vi "SyncronousLockin_single.vi"(4 "Lock-in settings":T1={"Averaging period, s"=0.0, "Output Representation"=enum."Real/Imaginary", "Output value"=enum."RMS", "Phase delay, points"=0} {"Averaging period, s" format="%#_6p"}, 5 "Raw points to average":i32, 6 "First chunk?":bool, 7 "CH name                          points   phase":T2, 8 "error in (no error)":errorcluster, 11 "Data":waveform(dbl)={"t0"=timestamp(0 s since 1904-01-01), "dt"=0.0, "Y"=[]}) -> (0 "error out":errorcluster, 3 "signal(s) out":waveform(dbl)[](array[waveform]))   [LabVIEW 2015]
uses:
  CH_name_pts_phase.ctl
  Syncronous Lockin Settings.ctl
  <vilib>/measure/NI_MABase.lvlib
panel:
  out "Waveform Graph":waveform(dbl)(graph)
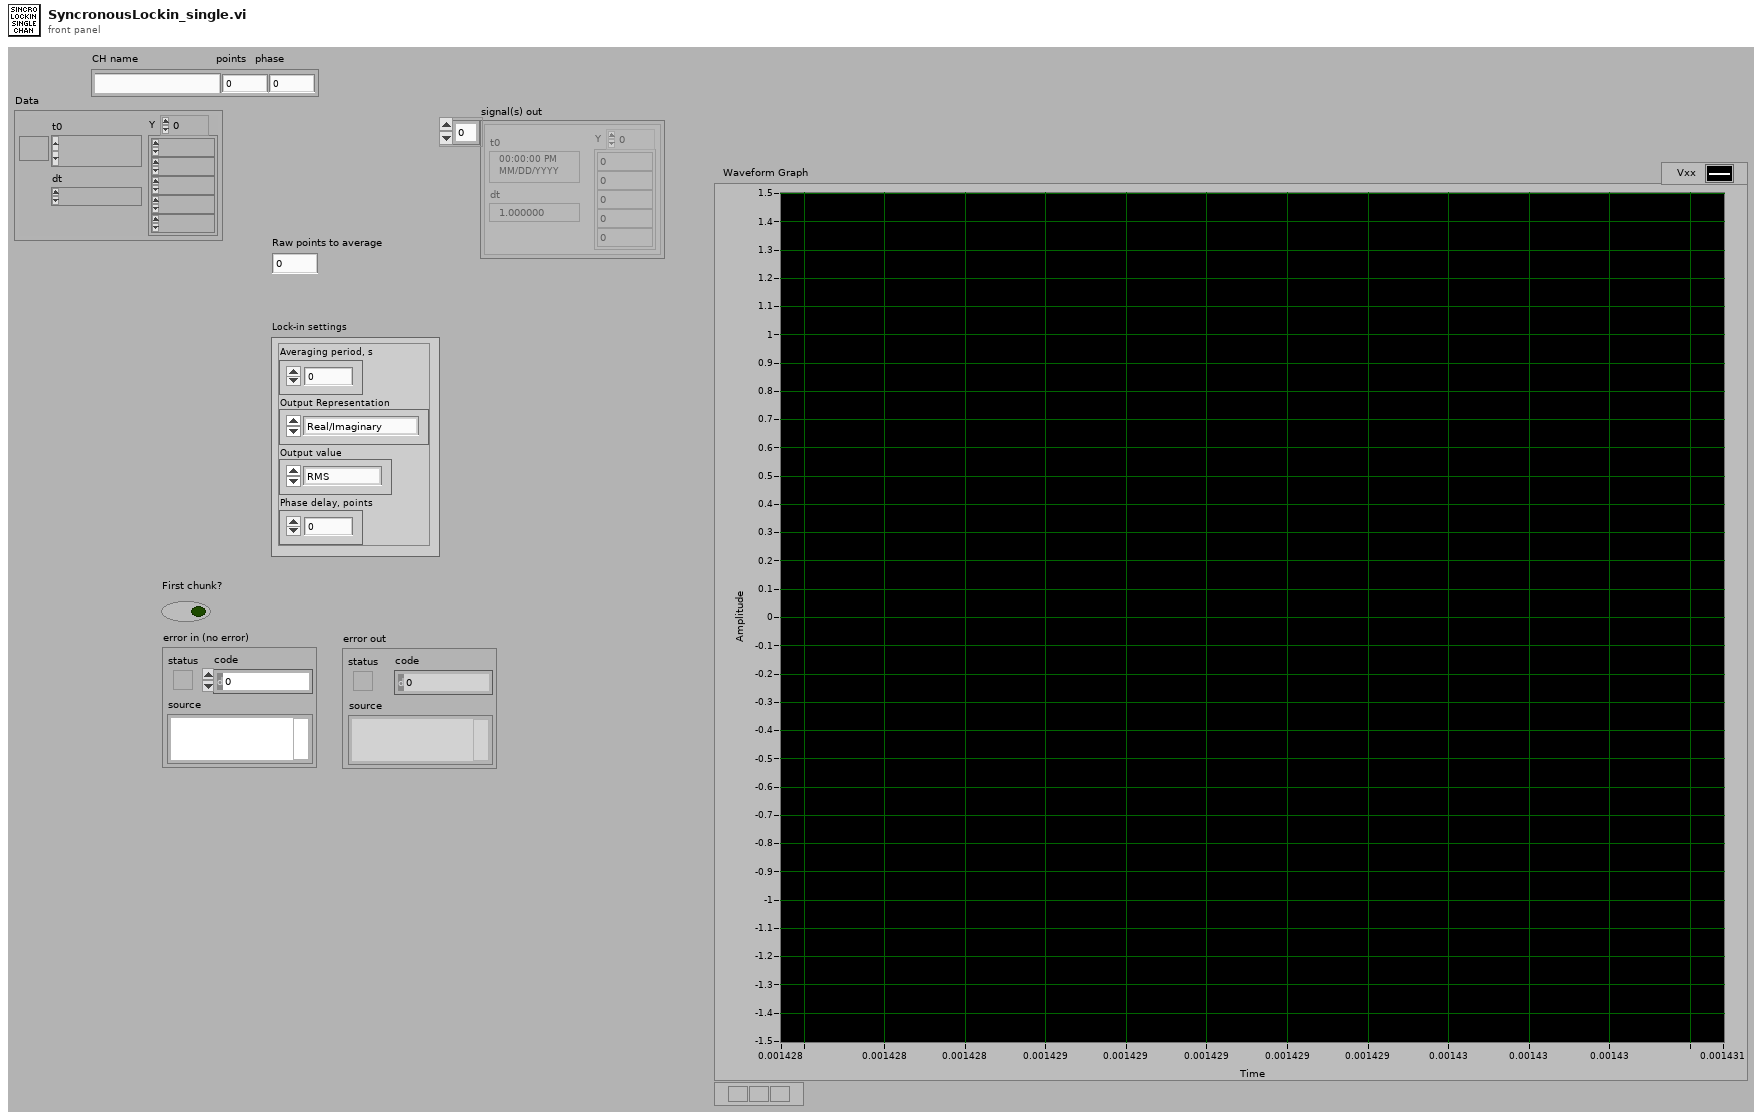
[diagram p1: front panel]
types:
  T1 = typedef "Syncronous Lockin Settings.ctl" = cluster{"Averaging period, s":dbl, "Output Representation":enum16{"Real/Imaginary", "Polar"}, "Output value":enum16{"Amplitude", "RMS", "Peak-to-Peak"}, "Phase delay, points":i32}
  T2 = typedef "CH_name_pts_phase.ctl" = cluster{"Channel":string, "pts per sine wave":i32, "Phase":dbl}
  T3 = enum16{"coerce", "linear", "spline", "Min-Max", "Average"}
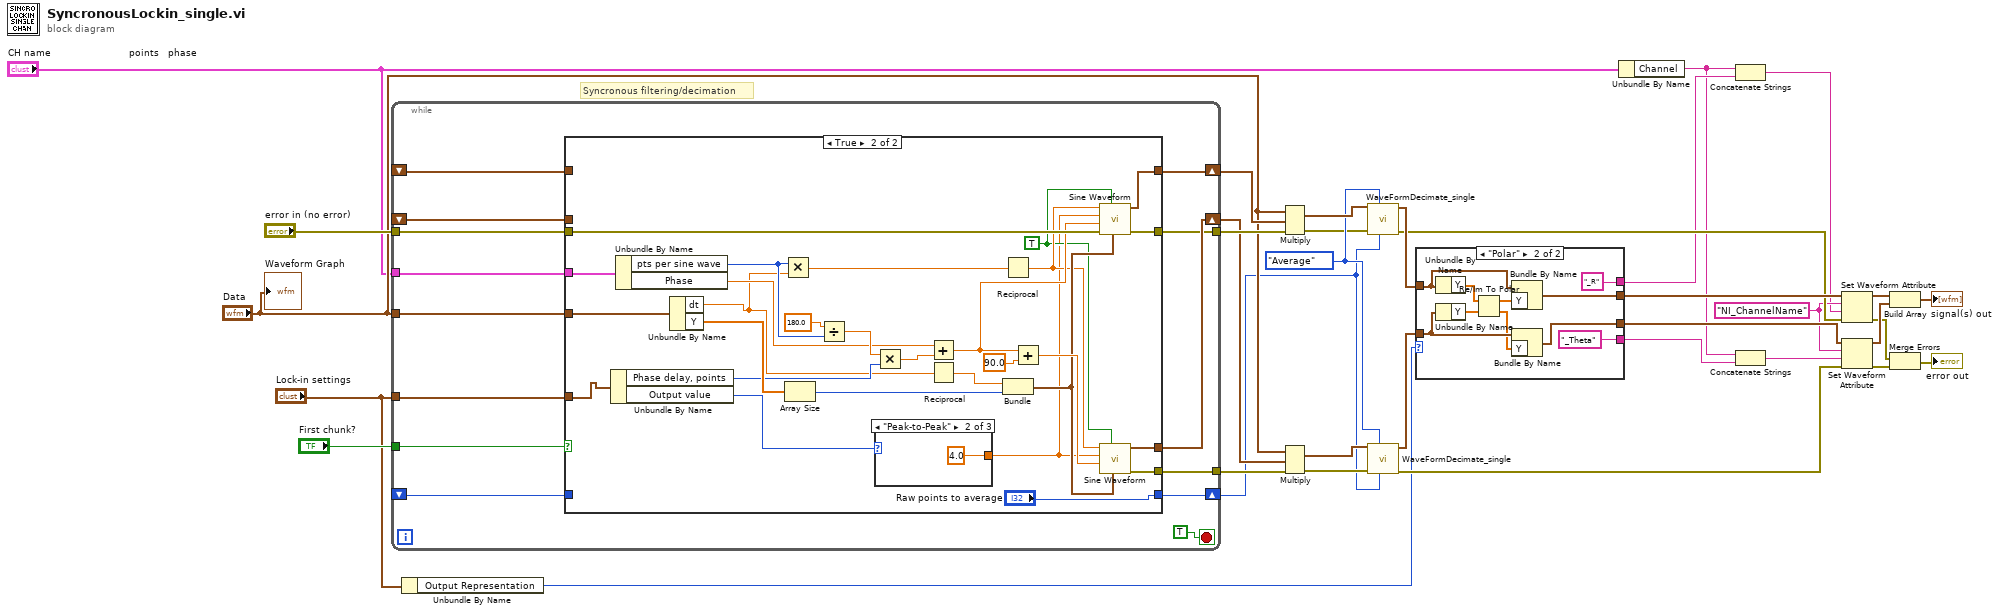
[diagram p0: block diagram]
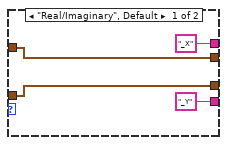
[diagram p2: hidden frame]
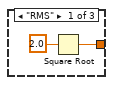
[diagram p4: hidden frame]
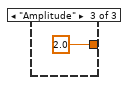
[diagram p5: hidden frame]
diagram:
  w10 = "NI_ChannelName" ("name")
  w24 = T3."Average" ("Plot interpolation")
  # "Syncronous filtering/decimation"
  n1 = while {
    tunnel: "Data" -> [w46]
    tunnel: "error in (no error)" -> [w45]
    tunnel: [w40] -> w33
    shift-right: [w48] -> w31
    shift-left: _ -> [w41]
    shift-right: [w47] -> w30
    shift-left: _ -> [w42]
    tunnel: "First chunk?" -> [w43]
    tunnel: [w39] -> w22
    tunnel: "CH name                          points   phase" -> [w38]
    tunnel: "Lock-in settings" -> [w37]
    shift-right: [w36] -> w3
    shift-left: _ -> [w35]
    stop <- TRUE stop-if-true
    n2 = case shown="True" w43 {
      tunnel: [w51 w79] -> w48
      tunnel: [w52 w78] -> w47
      tunnel: w46 -> [_ w61]
      tunnel: w45 -> [w50 w72]
      tunnel: [w50 w71] -> w39
      tunnel: w42 -> [w52 _]
      tunnel: w41 -> [w51 _]
      tunnel: [w50 w62] -> w40
      tunnel: w38 -> [_ w55]
      tunnel: w37 -> [_ w54]
      tunnel: [w49 "Raw points to average"] -> w36
      tunnel: w35 -> [w49 _]
      frame False {
      }
      frame True {
        w65 = TRUE ("reset signal")
        n3 = Unbundle By Name(w54) -> ("Phase delay, points"=w58:i32, "Output value"=w57:enum16{"Amplitude", "RMS", "Peak-to-Peak"})
        n4 = Unbundle By Name(w55) -> ("pts per sine wave"=w59:i32, "Phase"=w60:dbl)
        n5 = Unbundle By Name(w61) -> ("dt"=w56:dbl, "Y"=w75:dbl[])
        n6 = Multiply(x=w59, y=w56) -> (x*y=w69:dbl)
        n7 = Array Size(array=w75) -> (size(s)=w76:i32)
        n8 = Divide(x=180.0, y=w59) -> (x/y=w67:dbl)
        n9 = Multiply(x=w67, y=w58) -> (x*y=w66:dbl)
        n10 = case shown="\"Peak-to-Peak\"" w57 {
          tunnel: [w81 4.0 ("1/x") 2.0 ("1/x")] -> w63
          frame "RMS" {
            n11 = Square Root(x=2.0 ("1/x")) -> (sqrt(x)=w81:dbl)
          }
          frame "Peak-to-Peak" {
          }
          frame "Amplitude" {
          }
        }
        n12 = Add(x=w60, y=w66) -> (x+y=w70:dbl)
        n13 = Reciprocal(x=w56) -> (1/x=w73:dbl)
        n14 = Reciprocal(x=w69) -> (1/x=w68:dbl)
        n15 = Bundle(w73, w76) -> (w74:cluster{dbl, i32})  [unwired: 1 out]
        n16 = Add(x=w70, y=90.0) -> (x+y=w77:dbl)
        n17 = call <vilib>:"Sine Waveform.vi"("sampling info"=w74, "reset signal"=w65, "error in (no error)"=w72, "phase"=w70, "amplitude"=w63, "frequency"=w68) -> ("error out"=w62:errorcluster, "signal out"=w78:waveform(dbl))  [unwired: 1 in, 3 out]
        n18 = call <vilib>:"Sine Waveform.vi"("sampling info"=w74, "reset signal"=w65, "phase"=w77, "amplitude"=w63, "frequency"=w68) -> ("error out"=w71:errorcluster, "signal out"=w79:waveform(dbl))  [unwired: 2 in, 3 out]
      }
    }
  }
  n19 = Unbundle By Name("Lock-in settings") -> ("Output Representation"=w1:enum16{"Real/Imaginary", "Polar"})
  n20 = Multiply(1:w30, 2:"Data", 4:w33) -> (0:w29:waveform(dbl), 3:w20:errorcluster)
  n21 = Multiply(1:w31, 2:"Data", 4:w22) -> (0:w27:waveform(dbl), 3:w21:errorcluster)
  n22 = call "WaveFormDecimate_single.vi"("Decimation factor"=w3, "Plot interpolation"=w24, "error in (no error)"=w20, "Waveform in"=w29) -> ("error out"=w19:errorcluster, "Waveform out"=w28:waveform(dbl))  [unwired: 6 in]
  n23 = call "WaveFormDecimate_single.vi"("Decimation factor"=w3, "Plot interpolation"=w24, "error in (no error)"=w21, "Waveform in"=w27) -> ("error out"=w14:errorcluster, "Waveform out"=w26:waveform(dbl))  [unwired: 6 in]
  n24 = case shown="\"Polar\"" w1 {
    tunnel: w28 -> [w88 w98]
    tunnel: w26 -> [w87 w97]
    tunnel: [w87 w96] -> w18
    tunnel: [w88 w95] -> w23
    tunnel: ["_X" ("format string") "_R" ("format string")] -> w9
    tunnel: ["_Y" ("format string") "_Theta" ("format string")] -> w7
    frame "Real/Imaginary", Default {
    }
    frame "Polar" {
      n25 = Unbundle By Name(w98) -> ("Y"=w93:dbl[])
      n26 = Unbundle By Name(w97) -> ("Y"=w92:dbl[])
      n27 = Re/Im To Polar(2:w92, 3:w93) -> (0:w90:dbl[], 1:w91:dbl[])
      n28 = Bundle By Name(cluster=w98, "Y"=w91) -> (w95:waveform(dbl))
      n29 = Bundle By Name(cluster=w97, "Y"=w90) -> (w96:waveform(dbl))
    }
  }
  n30 = Unbundle By Name("CH name                          points   phase") -> ("Channel"=w5:string)
  n31 = Concatenate Strings(w5, w9) -> (w8:string)
  n32 = Concatenate Strings(w5, w7) -> (w6:string)
  n33 = Set Waveform Attribute(4:w19, 5:w8, 6:w10, 7:w23) -> (0:w13:errorcluster, 3:w17:waveform(dbl))  [unwired: 1 out]
  n34 = Set Waveform Attribute(4:w14, 5:w6, 6:w10, 7:w18) -> (0:w12:errorcluster, 3:w16:waveform(dbl))  [unwired: 1 out]
  n35 = Build Array(w17, w16) -> (→"signal(s) out":waveform(dbl)[])
  n36 = Merge Errors(w13, w12) -> (→"error out":errorcluster)
  "Waveform Graph" <- "Data"
